vi "Build Installer G-CLI.vi"(8 "error in (no error)":errorcluster, 11 "PostBuildSupport in":refnum<class "PostBuildSupport.lvclass">) -> (0 "error out":errorcluster, 3 "PostBuildSupport out":refnum<class "PostBuildSupport.lvclass">)   [LabVIEW 2019, in "PostBuildSupport.lvclass"]
uses:
  PostBuildSupport.lvclass
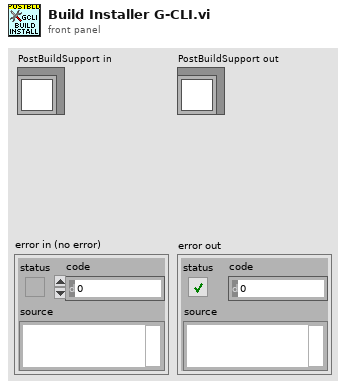
[diagram p1: front panel]
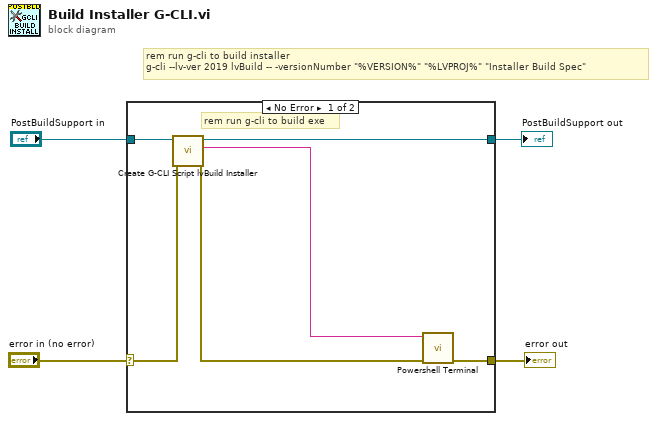
[diagram p0: block diagram]
diagram:
  # "rem run g-cli to build installer\ng-cli --lv-ver 2019 lvBuild -- -versionNumber \"%VERSION%\" \"%LVPROJ%\" \"Installer Build Spec\""
  n1 = case shown="No Error" "error in (no error)" {
    selector: "error in (no error)" -> [w9 w12]
    tunnel: "PostBuildSupport in" -> [w6 w11]
    tunnel: [w10 w12] -> w2
    tunnel: [w7 w11] -> w1
    frame No Error {
      # "rem run g-cli to build exe"
      n2 = call "Create G-CLI Script lvBuild Installer.vi"("error in (no error)"=w9, "PostBuildSupport in"=w6) -> ("error out"=w8:errorcluster, "command"=w5:string, "PostBuildSupport out"=w7:refnum<class "PostBuildSupport.lvclass">)  [unwired: 7 in]
      n3 = call "Powershell Terminal.vi"("error in (no error)"=w8, "StdIn"=w5) -> ("error out"=w10:errorcluster)  [unwired: 7 in, 2 out]
    }
    frame Error {
    }
  }
  "error out" <- w2
  "PostBuildSupport out" <- w1
